vi "LIA 4HF Decimators.vi"(5 "clock x 2":refnum<k21>, 7 "reset":bool, 9 "input valid":bool, 11 "data in":T1) -> (1 "output valid":bool, 3 "data out":T1)   [LabVIEW 2017]
uses:
  <instrlib>/_niInstr/DSP/v1/Shared/Public/IQ Data.ctl
  <instrlib>/_niInstr/DSP/v1/FPGA/Public/Sub VIs/HB Decimator/Halfband Decimator - IQ - 1 SPC - 2x OC.vi
  <instrlib>/_niInstr/DSP/v1/FPGA/niInstr DSP v1 FPGA.lvlib
  <instrlib>/_niInstr/DSP/v1/Shared/niInstr DSP v1 Shared.lvlib
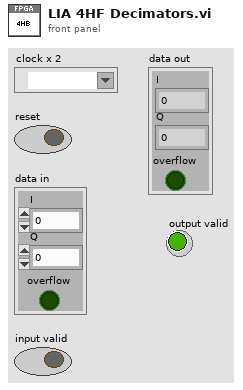
[diagram p1: front panel]
types:
  T1 = typedef "niInstr DSP v1 Shared.lvlib/IQ Data.ctl" = cluster{"I":fxp<+/-,18,1>, "Q":fxp<+/-,18,1>, "overflow":bool}
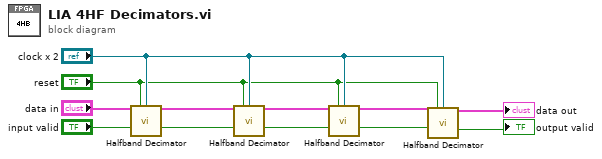
[diagram p0: block diagram]
diagram:
  n1 = call-poly <instrlib>:"Halfband Decimator.vi"("data in"="data in", "reset"="reset", "clock x 2"="clock x 2", "input valid"="input valid") -> ("data out"=w10:T1, "output valid"=w9:bool)  [unwired: 9 in, 1 out]
  n2 = call-poly <instrlib>:"Halfband Decimator.vi"("data in"=w10, "reset"="reset", "clock x 2"="clock x 2", "input valid"=w9) -> ("data out"=w7:T1, "output valid"=w3:bool)  [unwired: 9 in, 1 out]
  n3 = call-poly <instrlib>:"Halfband Decimator.vi"("data in"=w7, "reset"="reset", "clock x 2"="clock x 2", "input valid"=w3) -> ("data out"=w5:T1, "output valid"=w2:bool)  [unwired: 9 in, 1 out]
  n4 = call-poly <instrlib>:"Halfband Decimator.vi"("data in"=w5, "reset"="reset", "clock x 2"="clock x 2", "input valid"=w2) -> ("data out"=→"data out":T1, "output valid"=→"output valid":bool)  [unwired: 9 in, 1 out]
